vi "Mobility-Vt-Used Pts_Linear.vi"(5 "Width":dbl, 6 "Dielectric Const":dbl, 7 "Length":dbl, 8 "Vd":dbl, 9 "Dielectric (d)":dbl, 10 "Id Used":dbl[](array[numeric]), 11 "Vg Used":dbl[](array[numeric])) -> (1 "Capacitance":dbl, 2 "Vt":dbl, 3 "Mobility":dbl)   [LabVIEW 2012]
uses:
  <vilib>/Analysis/NI_AALPro.lvlib
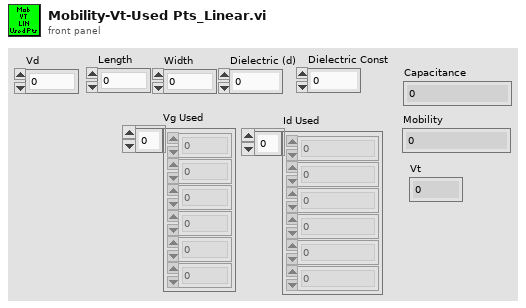
[diagram p1: front panel]
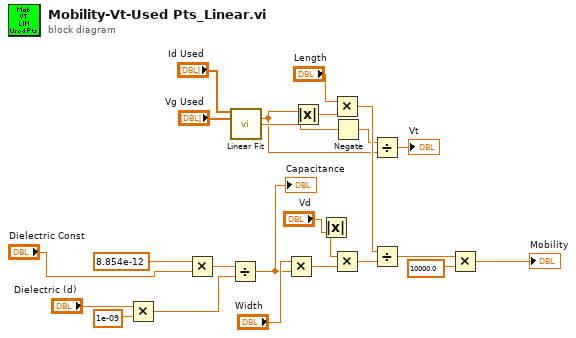
[diagram p0: block diagram]
diagram:
  n1 = Multiply(x="Dielectric (d)", y=1e-09) -> (x*y=w23:dbl)
  n2 = Multiply(x=8.854e-12, y="Dielectric Const") -> (x*y=w24:dbl)
  n3 = Divide(x=w24, y=w23) -> (x/y=w8:dbl)
  "Capacitance" <- w8
  n4 = call <vilib>:"Linear Fit.vi"("Y"="Id Used", "X"="Vg Used") -> ("slope"=w5:dbl, "intercept"=w9:dbl)  [unwired: 9 in, 3 out]
  n5 = Multiply(x="Width", y=w8) -> (x*y=w7:dbl)
  n6 = Absolute Value(x=w5) -> (abs(x)=w4:dbl)
  n7 = Absolute Value(x="Vd") -> (abs(x)=w1:dbl)
  n8 = Multiply(x="Length", y=w4) -> (x*y=w17:dbl)
  n9 = Multiply(x=w1, y=w7) -> (x*y=w6:dbl)
  n10 = Negate(x=w9) -> (-x=w10:dbl)
  n11 = Divide(x=w10, y=w5) -> (x/y=→"Vt":dbl)
  n12 = Divide(x=w17, y=w6) -> (x/y=w16:dbl)
  n13 = Multiply(x=w16, y=10000.0) -> (x*y=→"Mobility":dbl)
